vi "PanelOnTop.vi"(11 "VI Refnum":refnum<vi>) -> (0 "Error Out":errorcluster, 2 "Err":i32, 3 "Handler":u32)   [LabVIEW 2018]
uses:
  user32.dll
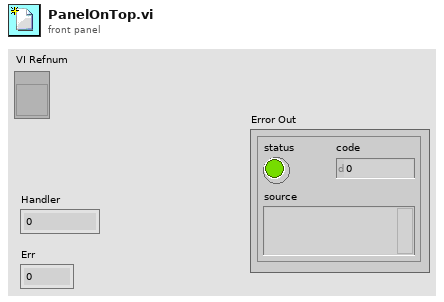
[diagram p1: front panel]
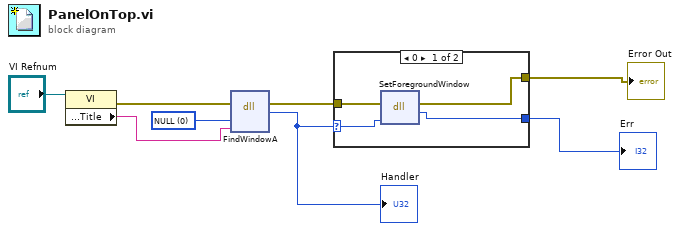
[diagram p0: block diagram]
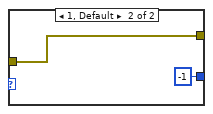
[diagram p2: hidden frame]
diagram:
  w8 = 0 items=["NULL"]
  n1 = property class="VI"(reference="VI Refnum") -> (error out=w5:errorcluster, "Front Panel.Title"=w6:string)  [unwired: 1 in, 1 out]
  n2 = dll-call lib="user32.dll" fn="FindWindowA" label="FindWindow"(error in=w5, "lpszClassName"=w8, "lpszWindowName"=w6) -> (error out=w1:errorcluster, "hWnd"=w4:u32)  [unwired: 3 in, 2 out]
  "Handler" <- w4
  n3 = case shown="0" w4 {
    selector: w4 -> [w10 _]
    tunnel: [w9 -1] -> w3
    tunnel: [w11 w13] -> w2
    tunnel: w1 -> [w12 w13]
    frame 0 {
      n4 = dll-call lib="user32.dll" fn="SetForegroundWindow"(error in=w12, "Handle"=w10) -> (error out=w11:errorcluster, "return type"=w9:i32)  [unwired: 3 in, 1 out]
    }
    frame 1, Default {
    }
  }
  "Err" <- w3
  "Error Out" <- w2
